vi "Exercises AM Demodulation.vi"(9 "载波幅度":dbl, 10 "载波频率":dbl, 11 "AM 调制信号 (时域)":waveform(dbl)) -> (3 "解调信号":waveform(dbl)(graph))   [LabVIEW 2015]
uses:
  <vilib>/measure/NI_MABase.lvlib
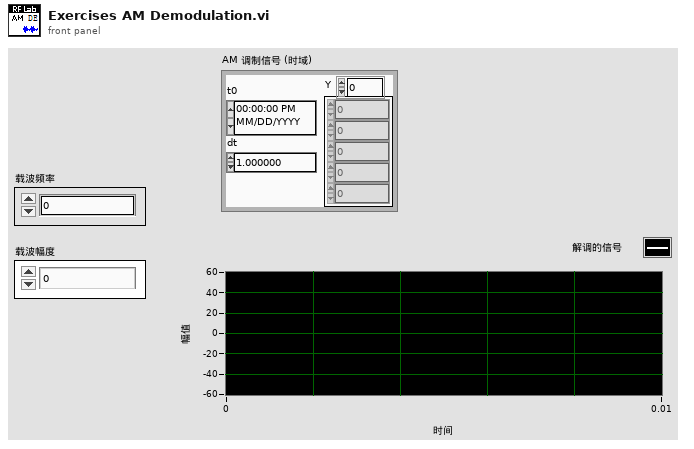
[diagram p1: front panel]
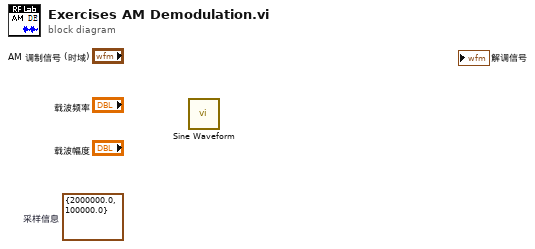
[diagram p0: block diagram]
diagram:
  (unwired) cluster{"Fs":dbl, "#s":dbl} {"Fs"=2000000.0, "#s"=100000.0}  # 采样信息
  n1 = call <vilib>:"Sine Waveform.vi"() -> ()  [unwired: 10 in, 2 out]
